vi "Add Item.vi"(8 "error in (no error)":errorcluster, 10 "Item to Add":string, 11 "StatusHistory in":refnum<class "StatusHistory.lvclass">) -> (0 "error out":errorcluster, 3 "StatusHistory out":refnum<class "StatusHistory.lvclass">)   [LabVIEW 2020, in "StatusHistory.lvclass"]
uses:
  StatusHistory.lvclass
  StatusHistory.lvclass/StatusHistory.ctl
  Read History Size.vi
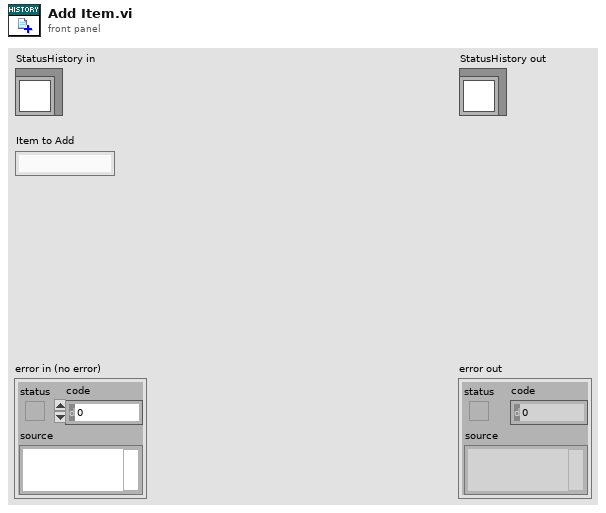
[diagram p1: front panel]
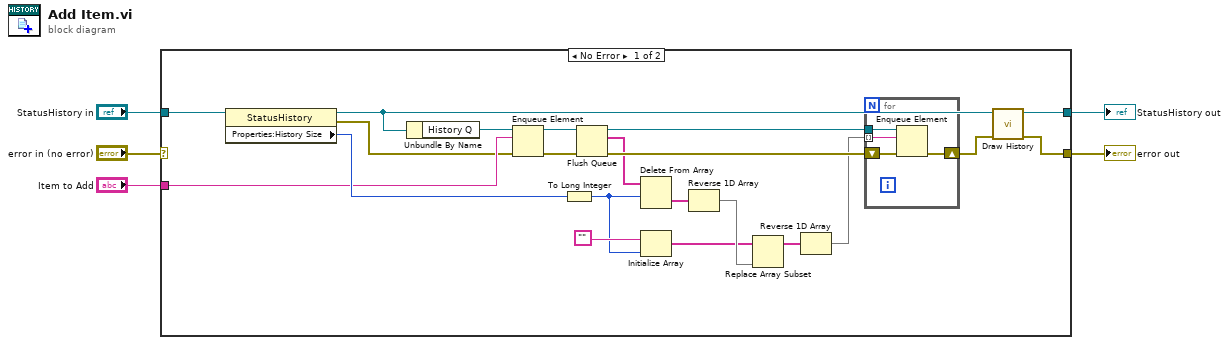
[diagram p0: block diagram]
diagram:
  n1 = case shown="No Error" "error in (no error)" {
    selector: "error in (no error)" -> [_ w32]
    tunnel: [w23 w32] -> w4
    tunnel: [w25 w31] -> w2
    tunnel: "StatusHistory in" -> [w26 w31]
    tunnel: "Item to Add" -> [w14 _]
    frame No Error {
      n2 = property class="StatusHistory"(reference=w26) -> (reference out=w22:refnum<class "StatusHistory.lvclass">, error out=w6:errorcluster, "Properties:History Size"=w18:u32)  [unwired: 1 in]
      n3 = Unbundle By Name(w22) -> ("History Q"=w16:refnum<queue>)
      n4 = Enqueue Element(queue=w16, element=w14, error in (no error)=w6) -> (queue out=w15:refnum<queue>, error out=w17:errorcluster)  [unwired: 1 in, 1 out]
      n5 = To Long Integer(number=w18) -> (32bit integer=w12:i32)
      n6 = Flush Queue(queue=w15, error in (no error)=w17) -> (queue out=w19:refnum<queue>, remaining elements=w13:string[], error out=w20:errorcluster)
      n7 = Delete From Array(array=w13, length=w12) -> (deleted portion=w11:string[])  [unwired: 1 in, 1 out]
      n8 = Initialize Array("", w12) -> (w9:string[])
      n9 = Reverse 1D Array(array=w11) -> (reversed array=w10:string[])
      n10 = Replace Array Subset(array=w9, new element=w10) -> (w8:string[])  [unwired: 1 in]
      n11 = Reverse 1D Array(array=w8) -> (reversed array=w7:string[])
      n12 = for {
        tunnel: w19 -> [w28]
        shift-right: [w30] -> w24
        shift-left: w20 -> [w29]
        tunnel: w7 -> [w27] mode=indexing
        n13 = Enqueue Element(queue=w28, element=w27, error in (no error)=w29) -> (error out=w30:errorcluster)  [unwired: 1 in, 2 out]
      }
      n14 = call "Draw History.vi"("error in (no error)"=w24, "StatusHistory in"=w22) -> ("error out"=w23:errorcluster, "StatusHistory out"=w25:refnum<class "StatusHistory.lvclass">)  [unwired: 8 in]
    }
    frame Error {
    }
  }
  "error out" <- w4
  "StatusHistory out" <- w2
